vi "Remove Cama from string input.vi"(11 "String in":string) -> (3 "string out":string)   [LabVIEW 2020]
uses:
  <vilib>/Utility/error.llb/whitespace.ctl
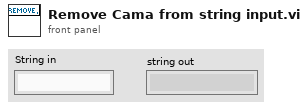
[diagram p1: front panel]
types:
  T1 = typedef "whitespace.ctl" = u16
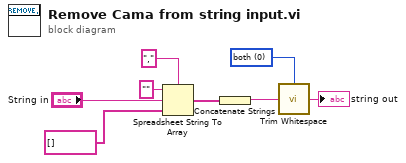
[diagram p0: block diagram]
diagram:
  w2 = T1 0 items=["both", "start of string", "end of string"] ("location (both)")
  n1 = Spreadsheet String To Array(delimiter (Tab)=",", format string="", spreadsheet string="String in", array type (2D Dbl)=string[] []) -> (array=w4:string[])
  n2 = Concatenate Strings(w4) -> (w3:string)
  n3 = call <vilib>:"Trim Whitespace.vi"("string"=w3, "location (both)"=w2) -> ("trimmed string"=→"string out":string)
